vi "ramp_pattern.vi"(8 "start":i32, 11 "end":i32) -> (3 "schodki":dbl[](array[numeric]))   [LabVIEW 2020]
doc: "ramp pattern"
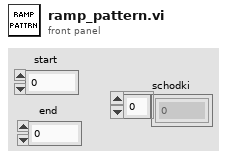
[diagram p1: front panel]
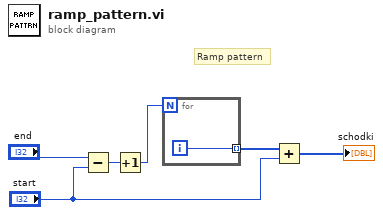
[diagram p0: block diagram]
diagram:
  # "Ramp pattern"
  n1 = Subtract(x="end", y="start") -> (x-y=w6:i32)
  n2 = Increment(x=w6) -> (x+1=w5:i32)
  n3 = for {
    N: w5 -> [_]
    tunnel: [w7] -> w4 mode=indexing
    i -> [w7]
  }
  n4 = Add(x=w4, y="start") -> (x+y=→"schodki":i32[])
